vi "NIManagement.vi"() -> (0 "error out":errorcluster, 1 "NI2":tag, 2 "NI1":tag, 4 "NI3":tag)   [LabVIEW 2017]
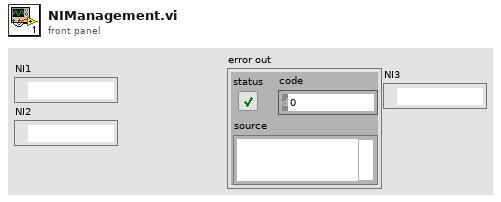
[diagram p1: front panel]
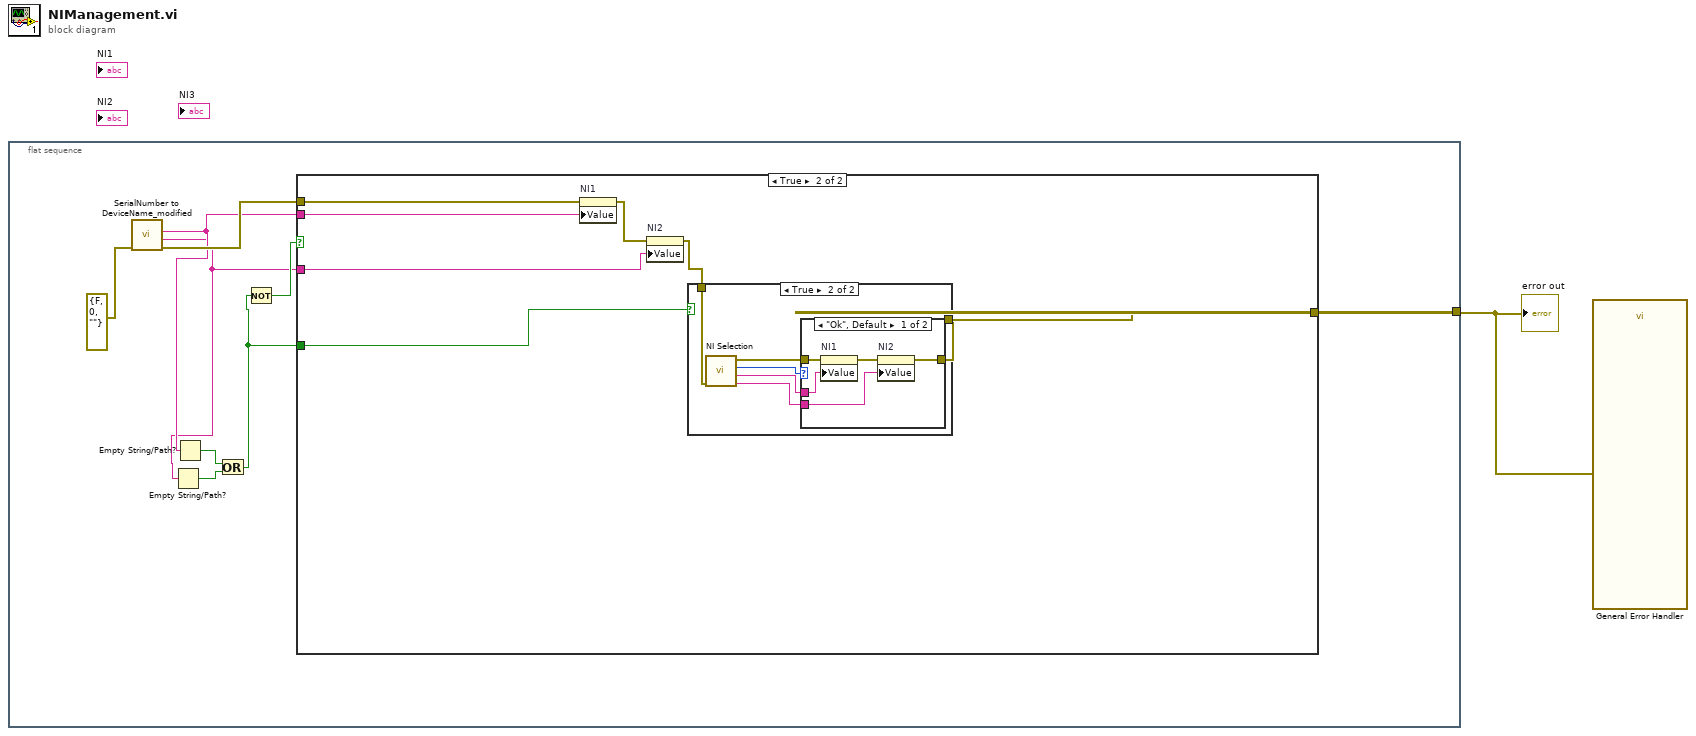
[diagram p0: block diagram]
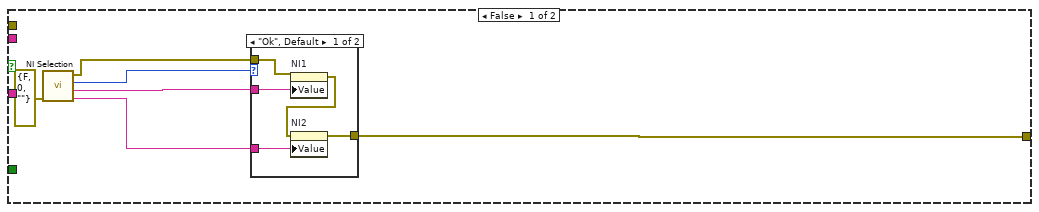
[diagram p2: hidden frame]
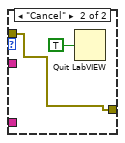
[diagram p3: hidden frame]
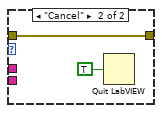
[diagram p5: hidden frame]
diagram:
  n1 = flat-sequence {
    tunnel: [w10] -> w1
    frame #0 {
      n2 = call "SerialNumber to DeviceName_modified.vi"("error in (no error)"=errorcluster {"status"=FALSE, "code"=0, "source"=""}) -> ("error out"=w8:errorcluster, "NI2 Device Name"=w2:tag, "NI1 Device Name"=w3:tag)  [unwired: 8 in]
      n3 = Empty String/Path?(string/path=w2) -> (empty?=w7:bool)
      n4 = Empty String/Path?(string/path=w3) -> (empty?=w6:bool)
      n5 = Or(x=w6, y=w7) -> (x .or. y?=w4:bool)
      n6 = Not(x=w4) -> (.not. x?=w5:bool)
      n7 = case shown="True" w5 {
        tunnel: [w11 w28] -> w10
        tunnel: w8 -> [_ w27]
        tunnel: w4 -> [_ w26]
        tunnel: w3 -> [_ w25]
        tunnel: w2 -> [_ w24]
        frame False {
          n8 = call "NI Selection.vi"("error in (no error)"=errorcluster {"status"=FALSE, "code"=0, "source"=""}) -> ("NI 2"=w14:tag, "NI 1"=w15:tag, "Ok/Cancel"=w16:enum16{"Ok", "Cancel"}, "error out"=w13:errorcluster)  [unwired: 6 in]
          n9 = case shown="\"Ok\", Default" w16 {
            tunnel: w15 -> [w21 _]
            tunnel: w14 -> [w20 _]
            tunnel: w13 -> [w19 w22]
            tunnel: [w17 w22] -> w11
            frame "Ok", Default {
              n10 = property on="NI1" class="DAQmxName"(error in=w19, "Value"=w21) -> (error out=w18:errorcluster)  [unwired: 1 in, 1 out]
              n11 = property on="NI2" class="DAQmxName"(error in=w18, "Value"=w20) -> (error out=w17:errorcluster)  [unwired: 1 in, 1 out]
            }
            frame "Cancel" {
              n12 = Quit LabVIEW(quit? (T)=TRUE) -> ()
            }
          }
        }
        frame True {
          n13 = property on="NI1" class="DAQmxName"(error in=w27, "Value"=w25) -> (error out=w30:errorcluster)  [unwired: 1 in, 1 out]
          n14 = property on="NI2" class="DAQmxName"(error in=w30, "Value"=w24) -> (error out=w29:errorcluster)  [unwired: 1 in, 1 out]
          n15 = case shown="True" w26 {
            tunnel: [w31 w33] -> w28
            tunnel: w29 -> [w31 w32]
            frame False {
            }
            frame True {
              n16 = call "NI Selection.vi"("error in (no error)"=w32) -> ("NI 2"=w35:tag, "NI 1"=w36:tag, "Ok/Cancel"=w37:enum16{"Ok", "Cancel"}, "error out"=w34:errorcluster)  [unwired: 6 in]
              n17 = case shown="\"Ok\", Default" w37 {
                tunnel: w36 -> [w42 _]
                tunnel: w35 -> [w41 _]
                tunnel: w34 -> [w38 w43]
                tunnel: [w39 w43] -> w33
                frame "Ok", Default {
                  n18 = property on="NI1" class="DAQmxName"(error in=w38, "Value"=w42) -> (error out=w40:errorcluster)  [unwired: 1 in, 1 out]
                  n19 = property on="NI2" class="DAQmxName"(error in=w40, "Value"=w41) -> (error out=w39:errorcluster)  [unwired: 1 in, 1 out]
                }
                frame "Cancel" {
                  n20 = Quit LabVIEW(quit? (T)=TRUE) -> ()
                }
              }
            }
          }
        }
      }
    }
  }
  n21 = call <vilib>:"General Error Handler.vi"("error in (no error)"=w1) -> ()  [unwired: 10 in, 5 out]
  "error out" <- w1
